vi "Verify as Binary File.vi"(5 "Options":T1, 7 "Test VI (caller)":string, 8 "error in":errorcluster, 9 "Extension":string, 10 "Path to Binary File to Verify":path) -> (0 "error out":errorcluster, 1 "Failure Message":string, 2 "Passed?":bool)   [LabVIEW 2020, in "Approval Tests.lvlib"]
doc: "Performs an approval test.\n\nThe first call, the test passes and the test data is written to the approved file.\n\nOn subsequent runs the test data is compared to the contents of the approved file.\nIf it is a match, the test passes.\nIf it is not a match, the test fails and the test data is written to the actual file.\n\nAt the point the user can diff the approved and actual files and determine if they approve of the changes or not. If they approve, they replace the old approved file with the actual file. \n\nNOTE: You should keep the approved files in Source Code Control. You should ignore *.actual in your .gitignore file - there is no need to store those."
uses:
  Approval Tests.lvlib
  Options.ctl
  Reporter/Reporter.lvclass
  Printer/Printer.lvclass
  <vilib>/security/Message Digest/API/Instances/File/SHA-256 File Checksum.vi
  <vilib>/security/Message Digest/API/NI_Message Digest API.lvlib
  <vilib>/SourceControl/sccapi/SCCAPI VI Compare Options.ctl
  <vilib>/SourceControl/sccapi/NI_SCC.lvlib
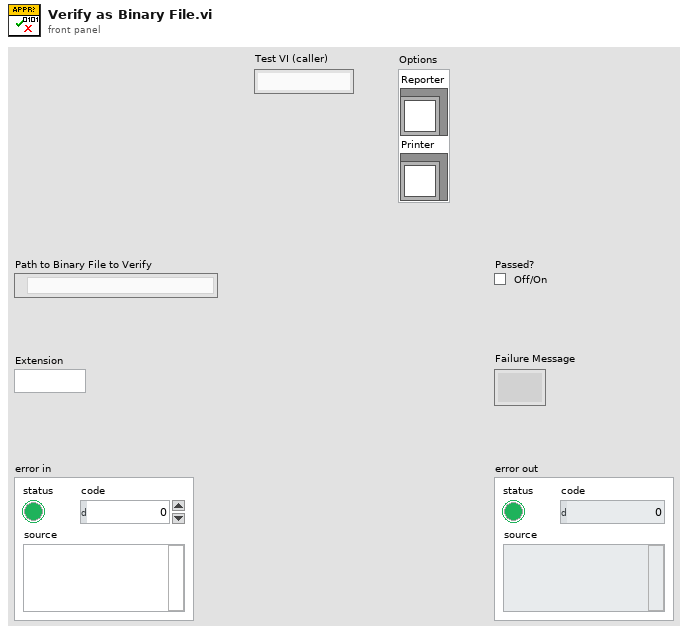
[diagram p1: front panel]
types:
  T1 = typedef "Approval Tests.lvlib/Options.ctl" = cluster{"Reporter":refnum<class "Reporter.lvclass">, "Printer":refnum<class "Printer.lvclass">}
  T2 = typedef "NI_SCC.lvlib/SCCAPI VI Compare Options.ctl" = cluster{"VI Attributes":bool, "Front Panel":bool, "FP position/size":bool, "Block Diagram":bool, "BD cosmetic":bool, "BD position/size":bool}
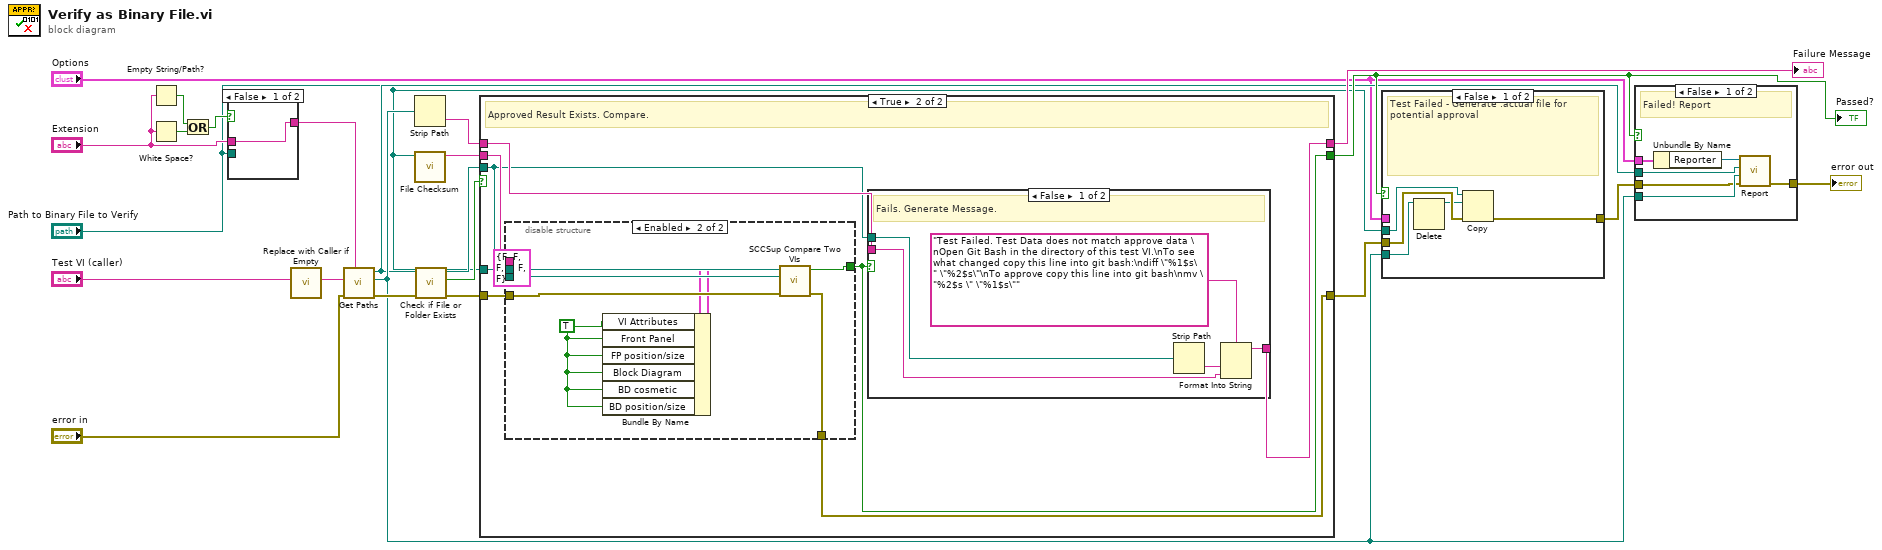
[diagram p0: block diagram]
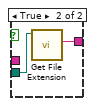
[diagram p2: hidden frame]
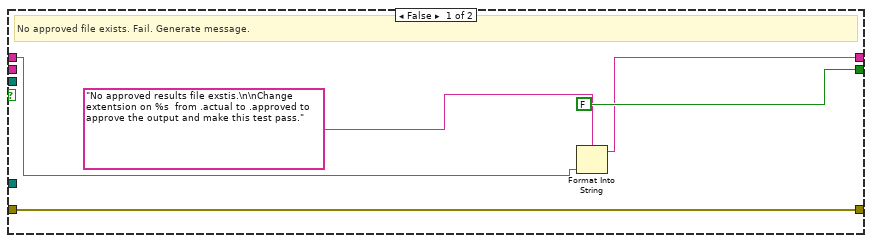
[diagram p5: hidden frame]
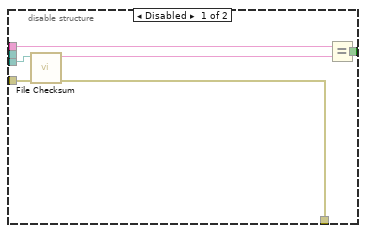
[diagram p6: hidden frame]
diagram:
  n1 = Empty String/Path?(string/path="Extension") -> (empty?=w6:bool)
  n2 = White Space?(1:"Extension") -> (0:w5:bool)
  n3 = Or(x=w6, y=w5) -> (x .or. y?=w4:bool)
  n4 = case shown="False" w4 {
    tunnel: "Path to Binary File to Verify" -> [_ w26]
    tunnel: [w24 w25] -> w3
    tunnel: "Extension" -> [w24 _]
    frame False {
    }
    frame True {
      n5 = call <vilib>:"Get File Extension.vi"("file"=w26) -> ("lowercase file extension"=w25:string)  [unwired: 6 in, 4 out]
    }
  }
  n6 = call "Replace with Caller if Empty.vi"("Test VI (caller) in"="Test VI (caller)") -> ("Test VI (caller) out"=w7:string)  [unwired: 10 in]
  n7 = call "Get Paths.vi"("Extension(txt)"=w3, "error in"="error in", "VI name"=w7) -> ("error out"=w23:errorcluster, "recived path"=w15:path, "approved path"=w14:path)  [unwired: 6 in]
  n8 = Strip Path(path=w15) -> (name=w17:string)  [unwired: 1 out]
  n9 = call-poly <vilib>:"File Checksum.vi"("path"="Path to Binary File to Verify") -> ("digest"=w9:string)  [unwired: 9 in, 1 out]
  n10 = call <vilib>:"Check if File or Folder Exists.vi"("error in (no error)"=w23, "path"=w14) -> ("error out"=w22:errorcluster, "file or folder exists?"=w19:bool, "dup path"=w20:path)  [unwired: 7 in]
  n11 = case shown="True" w19 {
    tunnel: w9 -> [_ w38]
    tunnel: [w31 w34] -> w21
    tunnel: w22 -> [w31 w35]
    tunnel: w20 -> [_ w33]
    tunnel: [FALSE ("Passed?") w39] -> w16
    tunnel: [w27 w37] -> w18
    tunnel: w17 -> [w29 w36]
    tunnel: "Path to Binary File to Verify" -> [_ w32]
    frame False {
      # "No approved file exists. Fail. Generate message."
      n12 = Format Into String(format string="No approved results file exstis.\n\nChange extentsion on %s  from .actual to .approved to approve the output and make this test pass.", w29) -> (resulting string=w27:string)  [unwired: 2 in, 1 out]
    }
    frame True {
      # "Approved Result Exists. Compare."
      n13 = disable-structure shown="Enabled" {
        disable-tunnel: [w45 w51] -> w39
        disable-tunnel: w38 -> [w44 _]
        disable-tunnel: w35 -> [w43 w53]
        disable-tunnel: [w42 w52] -> w34
        disable-tunnel: w33 -> [w40 w49]
        disable-tunnel: w32 -> [_ w50]
        frame Disabled {
          n14 = call-poly <vilib>:"File Checksum.vi"("error in"=w43, "path"=w40) -> ("error out"=w42:errorcluster, "digest"=w41:string)  [unwired: 8 in]
          n15 = Equal?(x=w44, y=w41) -> (x = y?=w45:bool)
        }
        frame Enabled {
          w46 = TRUE
          n16 = Bundle By Name(cluster=T2 {"VI Attributes"=FALSE, "Front Panel"=FALSE, "FP position/size"=FALSE, "Block Diagram"=FALSE, "BD cosmetic"=FALSE, "BD position/size"=FALSE} ("compare options"), "VI Attributes"=w46, "Front Panel"=w46, "FP position/size"=w46, "Block Diagram"=w46, "BD cosmetic"=w46, "BD position/size"=w46) -> (w47:T2)
          n17 = call <vilib>:"SCCSup Compare Two VIs.vi"("compare options"=w47, "error in (no error)"=w53, "Second VI"=w49, "First VI"=w50) -> ("error out"=w52:errorcluster, "Same?"=w51:bool)  [unwired: 5 in, 1 out]
        }
      }
      n18 = case shown="False" w39 {
        tunnel: [w58 _] -> w37
        tunnel: w33 -> [w55 _]
        tunnel: w36 -> [w54 _]
        frame False {
          # "Fails. Generate Message."
          n19 = Strip Path(path=w55) -> (name=w56:string)  [unwired: 1 out]
          n20 = Format Into String(format string="Test Failed. Test Data does not match approve data \nOpen Git Bash in the directory of this test VI.\nTo see what changed copy this line into git bash:\ndiff \"%1$s\" \"%2$s\"\nTo approve copy this line into git bash\nmv \"%2$s \" \"%1$s\"", w56, w54) -> (resulting string=w58:string)  [unwired: 2 in, 1 out]
        }
        frame True {
          # "Passes. No Message Needed.."
        }
      }
    }
  }
  "Passed?" <- w16
  "Failure Message" <- w18
  n21 = case shown="False" w16 {
    tunnel: w21 -> [w62 w64]
    tunnel: [w61 w64] -> w12
    tunnel: w15 -> [w63 _]
    tunnel: "Path to Binary File to Verify" -> [w59 _]
    tunnel: "Options" -> [_ _]
    frame False {
      # "Test Failed - Generate .actual file for potential approval"
      n22 = Delete(path (use dialog)=w63) -> (deleted path=w60:path)  [unwired: 4 in, 2 out]
      n23 = Copy(8:w62, 10:w60, 11:w59) -> (0:w61:errorcluster)  [unwired: 2 in, 2 out]
    }
    frame True {
      # "Passed - no need for .actual file"
    }
  }
  n24 = case shown="False" w16 {
    tunnel: w15 -> [w69 _]
    tunnel: w14 -> [w70 _]
    tunnel: w12 -> [w68 w71]
    tunnel: [w67 w71] -> w11
    tunnel: "Options" -> [w66 _]
    frame False {
      # "Failed! Report"
      n25 = Unbundle By Name(w66) -> ("Reporter"=w65:refnum<class "Reporter.lvclass">)
      n26 = call-dynamic "Report.vi"("error in (no error)"=w68, "Received"=w69, "Approved"=w70, "Reporter in"=w65) -> ("error out"=w67:errorcluster)  [unwired: 6 in, 1 out]
    }
    frame True {
      # "Passed - Nothing to Report"
    }
  }
  "error out" <- w11
